vi "load limit line.vi"(8 "Input trace 2D array":dbl[][](array[numeric]), 11 "Input limit 2D array":dbl[][](array[numeric])) -> (0 "Output Limit Cluster":cluster{"xi used":dbl[], "yi":dbl[]}, 3 "Output limit 2D array":dbl[][](array[numeric]))   [LabVIEW 2016]
doc: "this SubVI load limit line onto the XY graph"
uses:
  <vilib>/gmath/NI_Gmath.lvlib
panel:
  out "Number of points":i32
  out "XY Graph":cluster{"xi used":dbl[], "yi":dbl[]}(graph)
  out "Trace Frequency":dbl[](array[numeric])
  out "Trace amplitude":dbl[](array[numeric])
  out "Limit Frequency":dbl[](array[numeric])
  out "Limit Value":dbl[](array[numeric])
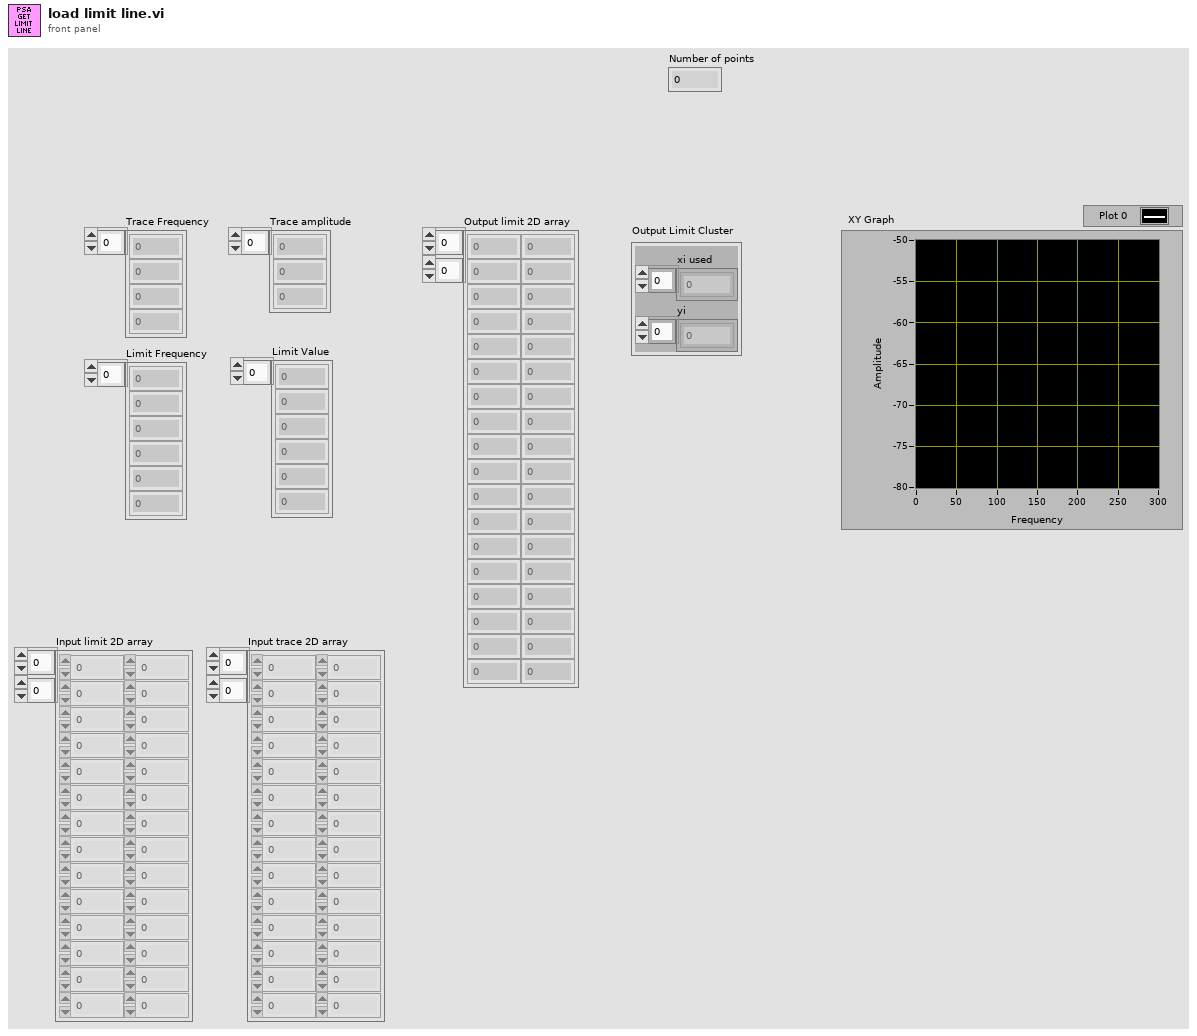
[diagram p1: front panel]
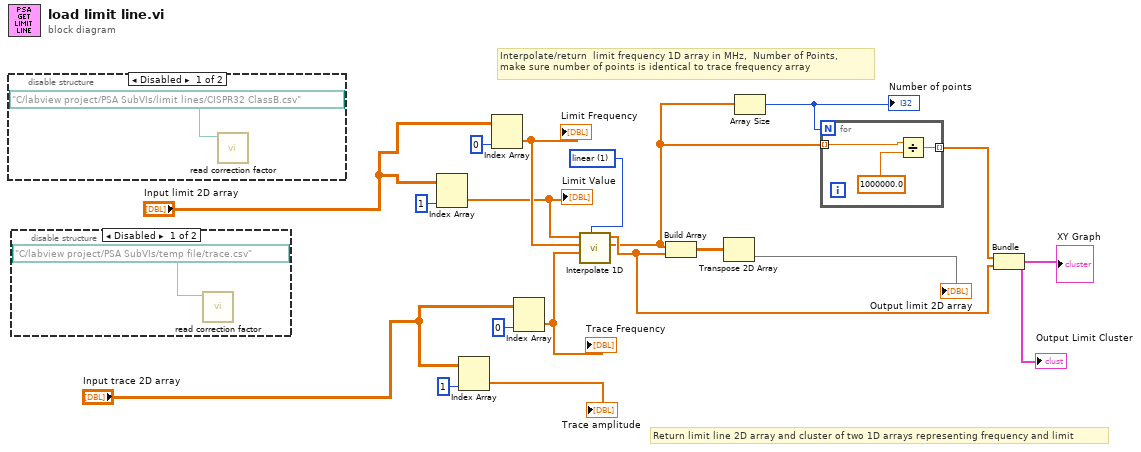
[diagram p0: block diagram]
diagram:
  w6 = 1 items=["nearest", "linear", "spline", "cubic Hermite", "Lagrange"] ("method")
  # "Interpolate/return  limit frequency 1D array in MHz,  Number of Points,\nmake sure number of points is identical to trace frequency array"
  # "Return limit line 2D array and cluster of two 1D arrays representing frequency and limit"
  n1 = disable-structure shown="Disabled" {
    frame Disabled {
      n2 = call "read correction factor.vi"("Path"=path "C:/labview project/PSA SubVIs/limit lines/CISPR32 ClassB.csv") -> ()  [unwired: 7 in, 4 out]
    }
    frame Enabled {
    }
  }
  n3 = disable-structure shown="Disabled" {
    frame Disabled {
      n4 = call "read correction factor.vi"("Path"=path "C:/labview project/PSA SubVIs/temp file/trace.csv") -> ()  [unwired: 7 in, 4 out]
    }
    frame Enabled {
    }
  }
  n5 = Index Array(array="Input limit 2D array", index (col)=1 ("disabled index (col)")) -> (element=w11:dbl[])  [unwired: 1 in]
  "Limit Value" <- w11
  n6 = Index Array(array="Input trace 2D array", index (col)=1 ("disabled index (col)")) -> (element=→"Trace amplitude":dbl[])  [unwired: 1 in]
  n7 = Index Array(array="Input limit 2D array", index (col)=0 ("disabled index (col)")) -> (element=w12:dbl[])  [unwired: 1 in]
  "Limit Frequency" <- w12
  n8 = Index Array(array="Input trace 2D array", index (col)=0 ("disabled index (col)")) -> (element=w13:dbl[])  [unwired: 1 in]
  "Trace Frequency" <- w13
  n9 = call <vilib>:"Interpolate 1D.vi"("method"=w6, "xi"=w13, "X"=w12, "Y"=w11) -> ("xi used"=w4:dbl[], "yi"=w8:dbl[])  [unwired: 5 in, 1 out]
  n10 = Build Array(w4, w8) -> (w9:dbl[][])
  n11 = Transpose 2D Array(2D array=w9) -> (transposed array=→"Output limit 2D array":dbl[][])
  n12 = Array Size(array=w4) -> (size(s)=w5:i32)
  "Number of points" <- w5
  n13 = for {
    N: w5 -> [_]
    tunnel: w4 -> [w22] mode=indexing
    tunnel: [w21] -> w3 mode=indexing
    n14 = Divide(x=w22, y=1000000.0) -> (x/y=w21:dbl)
  }
  n15 = Bundle(w3, "yi"=w8) -> (→"XY Graph" →"Output Limit Cluster":cluster{dbl[], "yi":dbl[]})  [unwired: 1 in]
